vi "Table Color Init.vi"(10 "Start Line":i16=1, 11 "Table in":refnum<vi>) -> ()   [LabVIEW 2011]
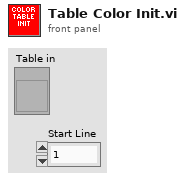
[diagram p1: front panel]
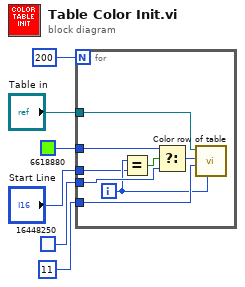
[diagram p0: block diagram]
diagram:
  n1 = for {
    N: 200 -> [_]
    tunnel: "Table in" -> [w14]
    tunnel: u32 16448250 -> [w10]
    tunnel: 11 -> [w13]
    tunnel: u32 6618880 -> [w11]
    tunnel: "Start Line" -> [w7]
    i -> [w8]
    n2 = Equal?(x=w8, y=w7) -> (x = y?=w12:bool)
    n3 = Select(t=w11, s=w12, f=w10) -> (s? t:f=w9:u32)
    n4 = call "Color row of table.vi"("Edit Line"=w8, "Number of Columns"=w13, "Color"=w9, "Table in"=w14) -> ()  [unwired: 7 in, 1 out]
  }
